vi "Send CMD_M1_2.vi"(5 "Speed (mm/s) M1":i32, 6 "SERVO ON CMD M1":bool, 8 "Home Calling M1":bool, 9 "Pokayoka":bool, 10 "Travel (mm)M1":i32, 11 "LCD Pressing Servo":T1) -> ()   [LabVIEW 2015]
uses:
  Galobal variable_TI.vi
  Project Setup/Globle Variable/GR_Servo.vi
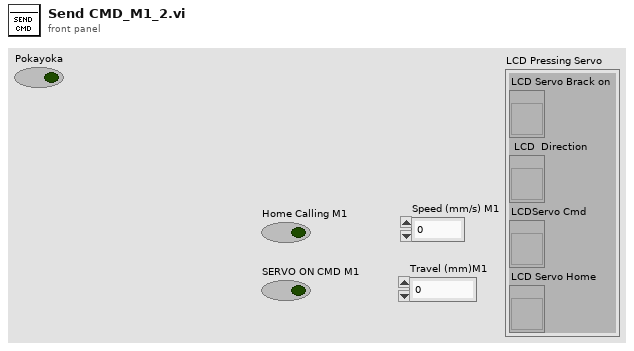
[diagram p1: front panel]
types:
  T1 = cluster{"LCD Servo Brack on":refnum<vi>, " LCD  Direction":refnum<vi>, "LCDServo Cmd":refnum<vi>, "LCD Servo Home":refnum<vi>}
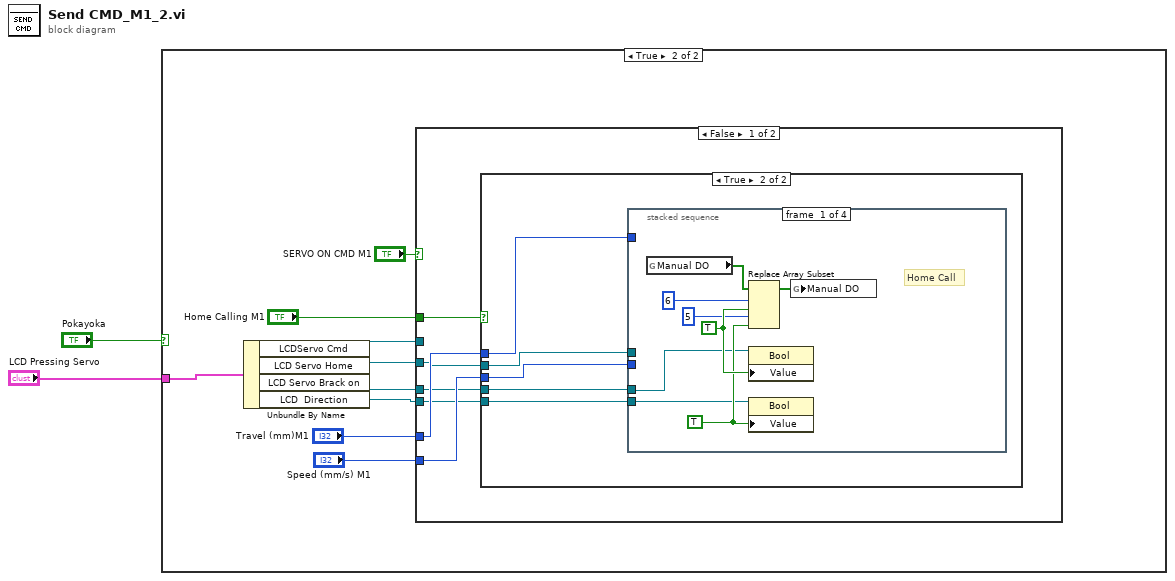
[diagram p0: block diagram]
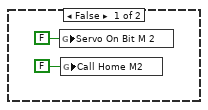
[diagram p3: hidden frame]
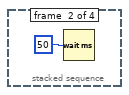
[diagram p4: hidden frame]
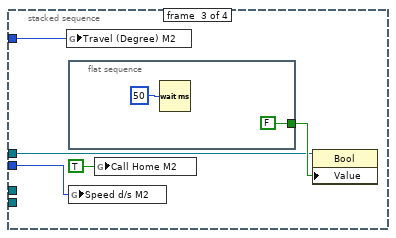
[diagram p5: hidden frame]
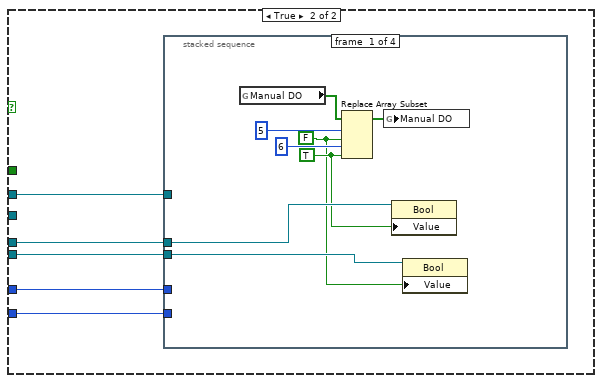
[diagram p7: hidden frame]
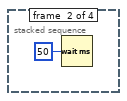
[diagram p8: hidden frame]
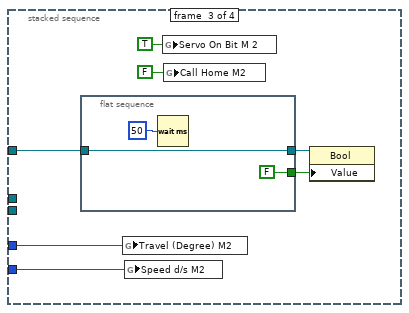
[diagram p9: hidden frame]
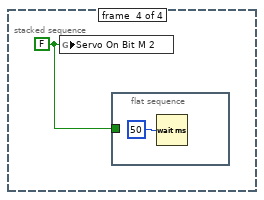
[diagram p10: hidden frame]
diagram:
  n1 = case shown="True" "Pokayoka" {
    tunnel: "LCD Pressing Servo" -> [_ w3]
    frame False {
    }
    frame True {
      n2 = Unbundle By Name(w3) -> ("LCDServo Cmd"=w4:refnum<vi>, "LCD Servo Home"=w5:refnum<vi>, "LCD Servo Brack on"=w7:refnum<vi>, "LCD  Direction"=w6:refnum<vi>)
      n3 = case shown="False" "SERVO ON CMD M1" {
        tunnel: "Speed (mm/s) M1" -> [w16 w45]
        tunnel: "Travel (mm)M1" -> [w15 w44]
        tunnel: "Home Calling M1" -> [w17 _]
        tunnel: w4 -> [_ w43]
        tunnel: w5 -> [w14 _]
        tunnel: w7 -> [w13 w42]
        tunnel: w6 -> [w12 w41]
        frame False {
          n4 = case shown="True" w17 {
            tunnel: w16 -> [_ w21]
            tunnel: w15 -> [_ w20]
            tunnel: w14 -> [_ w22]
            tunnel: w13 -> [_ w24]
            tunnel: w12 -> [_ w23]
            frame False {
              n5 = global write "GR_Servo.vi" "Servo On Bit M 2"(FALSE ("Servo On Bit")) -> ()
              n6 = global write "Galobal variable_TI.vi" "Call Home M2"(FALSE ("Call Home M1")) -> ()
            }
            frame True {
              n7 = stacked-sequence {
                tunnel: w24 -> [w25 _ _ _]
                tunnel: w23 -> [w26 _ _ _]
                tunnel: w22 -> [_ _ w36 _]
                tunnel: w21 -> [_ _ w35 _]
                tunnel: w20 -> [_ _ w34 _]
                frame #0 {
                  w28 = TRUE ("new element/subarray")
                  w30 = TRUE ("new element/subarray")
                  # "Home Call"
                  n8 = global read "Galobal variable_TI.vi" "Manual DO"() -> (w27:bool[])
                  n9 = Replace Array Subset(array=w27, new element #1=w30, index #1=6 ("index"), new element #2=w28, index #2=5 ("index")) -> (w32:bool[])
                  n10 = property class="Bool"(reference=w25, "Value"=w30) -> ()  [unwired: 1 in, 2 out]
                  n11 = property class="Bool"(reference=w26, "Value"=w28) -> ()  [unwired: 1 in, 2 out]
                  n12 = global write "Galobal variable_TI.vi" "Manual DO"(w32) -> ()
                }
                frame #1 {
                  n13 = Wait (ms)(milliseconds to wait=u32 50) -> ()  [unwired: 1 out]
                }
                frame #2 {
                  n14 = global write "GR_Servo.vi" "Travel (Degree) M2"(w34) -> ()
                  n15 = flat-sequence {
                    tunnel: [FALSE ("SERVO ON CMD M1")] -> w37
                    frame #0 {
                      n16 = Wait (ms)(milliseconds to wait=u32 50) -> ()  [unwired: 1 out]
                    }
                  }
                  n17 = global write "GR_Servo.vi" "Speed d/s M2"(w35) -> ()
                  n18 = global write "Galobal variable_TI.vi" "Call Home M2"(TRUE ("Call Home M1")) -> ()
                  n19 = property class="Bool"(reference=w36, "Value"=w37) -> ()  [unwired: 1 in, 2 out]
                }
                frame #3 {
                }
              }
            }
          }
        }
        frame True {
          n20 = stacked-sequence {
            tunnel: w45 -> [_ _ w61 _]
            tunnel: w44 -> [_ _ w60 _]
            tunnel: w43 -> [_ _ w57 _]
            tunnel: w42 -> [w49 _ _ _]
            tunnel: w41 -> [w48 _ _ _]
            frame #0 {
              w47 = TRUE ("new element/subarray")
              w46 = FALSE ("new element/subarray")
              n21 = global read "Galobal variable_TI.vi" "Manual DO"() -> (w50:bool[])
              n22 = Replace Array Subset(array=w50, new element #1=w46, index #1=5 ("index"), new element #2=w47, index #2=6 ("index")) -> (w53:bool[])
              n23 = global write "Galobal variable_TI.vi" "Manual DO"(w53) -> ()
              n24 = property class="Bool"(reference=w49, "Value"=w47) -> ()  [unwired: 1 in, 2 out]
              n25 = property class="Bool"(reference=w48, "Value"=w46) -> ()  [unwired: 1 in, 2 out]
            }
            frame #1 {
              n26 = Wait (ms)(milliseconds to wait=u32 50) -> ()  [unwired: 1 out]
            }
            frame #2 {
              n27 = flat-sequence {
                tunnel: [w63] -> w56
                tunnel: w57 -> [w63]
                tunnel: [FALSE ("SERVO ON CMD M1")] -> w55
                frame #0 {
                  n28 = Wait (ms)(milliseconds to wait=u32 50) -> ()  [unwired: 1 out]
                }
              }
              n29 = global write "GR_Servo.vi" "Travel (Degree) M2"(w60) -> ()
              n30 = global write "GR_Servo.vi" "Speed d/s M2"(w61) -> ()
              n31 = global write "GR_Servo.vi" "Servo On Bit M 2"(TRUE ("Servo On Bit")) -> ()
              n32 = global write "Galobal variable_TI.vi" "Call Home M2"(FALSE ("Call Home M1")) -> ()
              n33 = property class="Bool"(reference=w56, "Value"=w55) -> ()  [unwired: 1 in, 2 out]
            }
            frame #3 {
              w65 = FALSE ("Servo On Bit")
              n34 = global write "GR_Servo.vi" "Servo On Bit M 2"(w65) -> ()
              n35 = flat-sequence {
                tunnel: w65 -> [_]
                frame #0 {
                  n36 = Wait (ms)(milliseconds to wait=u32 50) -> ()  [unwired: 1 out]
                }
              }
            }
          }
        }
      }
    }
  }
